vi "Tusk Conversion.vi"(1 "Joystick Input":dbl) -> (0 "Encoder Value":dbl)   [LabVIEW 2017]
doc: "Takes a number, multiplies it by 4096 (one encoder rotation), divides it by 360 and multilies the quotient by 270."
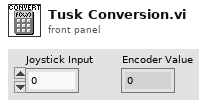
[diagram p1: front panel]
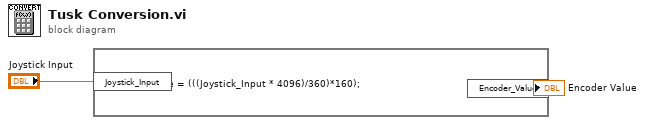
[diagram p0: block diagram]
diagram:
  n1 = formula code="Encoder_Value = (((Joystick_Input * 4096)/360)*160);"("Joystick_Input"="Joystick Input") -> ("Encoder_Value"=→"Encoder Value":dbl)
